vi "Global Parameters.vi"() -> ()   [LabVIEW 2015]
panel:
  in  "TCP ID":refnum<k5>
  out "TCP":bool
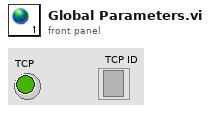
[diagram p1: front panel]
diagram:
